vi "Operator Actions Log.vi"() -> (3 "?":string)   [LabVIEW 2017]
uses:
  <vilib>/OPCUA/NI OPC UA Client.lvlib
panel:
  in  "Stop Log":bool
  out "Operator Actions Recording":bool
  out "Log Loop":i32
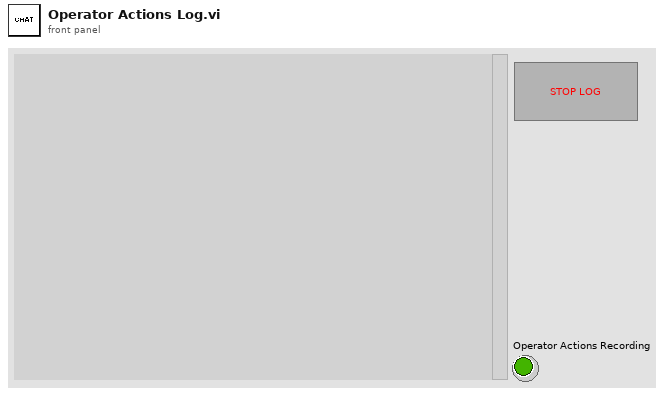
[diagram p1: front panel]
types:
  T1 = enum16{"open", "replace", "create", "open or create", "replace or create", "replace or create with confirmation"}
  T2 = typedef "OPC UA Client Refnum.ctl" = refnum<k21>
  T3 = typedef "Subscription ID.ctl" = u32
  T4 = typedef "Subscription Data Change.ctl" = cluster{"node ID":T5, " value":variant, "timestamp":timestamp, "data type":T6, "status code":T7}
  T5 = typedef "NodeId.ctl" = string
  T6 = typedef "Data Type.ctl" = u16
  T7 = typedef "OPC UA StatusCode.ctl" = u32
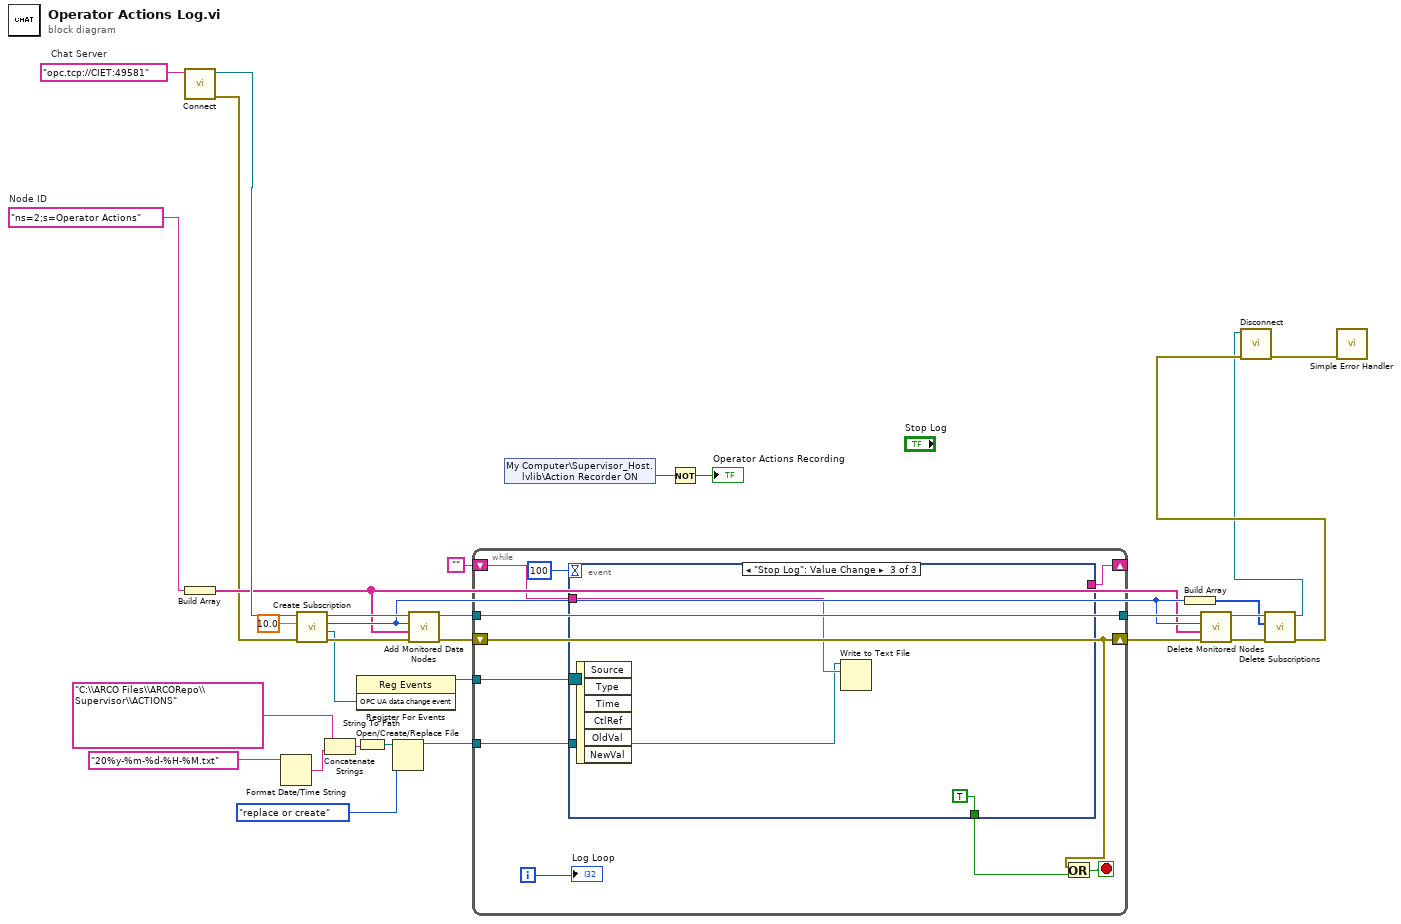
[diagram p0: block diagram]
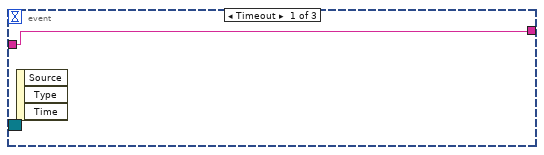
[diagram p2: hidden frame]
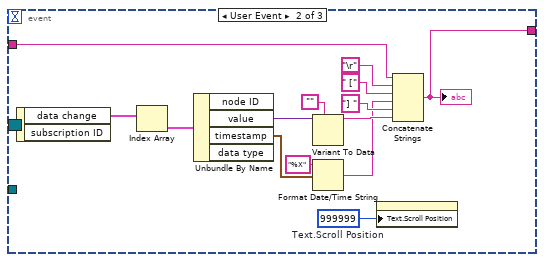
[diagram p3: hidden frame]
diagram:
  w15 = "ns=2;s=Operator Actions"  # Node ID
  w30 = "opc.tcp://CIET:49581"  # Chat Server
  n1 = call <vilib>:"Connect.vi"("server endpoint URL"=w30) -> ("error out"=w6:errorcluster, "OPC UA client refnum out"=w29:T2)  [unwired: 8 in, 1 out]
  n2 = Build Array(w15) -> (w14:string[])
  n3 = Format Date/Time String(time format string (%c)="20%y-%m-%d-%H-%M.txt") -> (date/time string=w10:string)  [unwired: 2 in]
  n4 = call <vilib>:"Create Subscription.vi"("error in (no error)"=w6, "publishing interval (1000 ms)"=10.0, "OPC UA client refnum in"=w29) -> ("error out"=w27:errorcluster, "OPC UA data change event"=w26:refnum<user-event>, "subscription ID out"=w18:T3, "OPC UA client refnum out"=w28:T2)  [unwired: 4 in, 1 out]
  n5 = Concatenate Strings("C:\\ARCO Files\\ARCORepo\\Supervisor\\ACTIONS", w10) -> (w8:string)
  n6 = register-events(w26) -> (reference out=w25:refnum<event-registration>)  [unwired: 2 in, 1 out]
  n7 = String To Path(string=w8) -> (path=w7:path)
  n8 = Open/Create/Replace File(file path (use dialog)=w7, operation (0:open)=T1."replace or create") -> (refnum out=w16:refnum<file>)  [unwired: 4 in, 2 out]
  n9 = call <vilib>:"Add Monitored Data Nodes.vi"("error in (no error)"=w27, "node IDs"=w14, "subscription ID in"=w18, "OPC UA client refnum in"=w28) -> ("error out"=w21:errorcluster, "OPC UA client refnum out"=w23:T2)  [unwired: 4 in, 2 out]
  n10 = while {
    tunnel: w25 -> [w41]
    shift-right: [w39] -> _
    shift-left: "" -> [w40]
    tunnel: w23 -> [w38]
    tunnel: [w38] -> w22
    tunnel: w16 -> [w37]
    shift-right: [w33] -> w5
    shift-left: w21 -> [w33]
    i -> [w36]
    stop <- w34 stop-if-true
    n11 = event shown="[2] \"Stop Log\": Value Change" {
      selector: w41 -> [_ _ _]
      dyn-events: _ -> [_ _ _]
      timeout: 100 -> [_ _ _]
      tunnel: w40 -> [w42 w45 w59]
      tunnel: [w42 w44 _] -> w39
      tunnel: w37 -> [_ _ w58]
      tunnel: [_ _ TRUE] -> w32
      event Timeout {
        n12 = event-data() -> ()  [unwired: 1 in, 3 out]
      }
      event User Event {
        w43 = u32 999999  # Text.Scroll Position
        n13 = event-data() -> ("data change"=w56:T4[])  [unwired: 1 in, 1 out]
        n14 = Index Array(array=w56) -> (element=w55:T4)  [unwired: 1 in]
        n15 = Unbundle By Name(w55) -> ("value"=w54:variant, "timestamp"=w52:timestamp)  [unwired: 2 out]
        n16 = Variant To Data(type="", Variant=w54) -> (data=w50:string)  [unwired: 1 in, 1 out]
        n17 = Format Date/Time String(time format string (%c)="%X", seconds (now)=w52) -> (date/time string=w48:string)  [unwired: 1 in]
        n18 = property class="Str"("Text.Scroll Position"=w43) -> ()  [unwired: 2 in, 2 out]
        n19 = Concatenate Strings(w45, "\r", " [", w48, "] ", w50) -> (w44:string)
        "?" <- w44
      }
      event "Stop Log": Value Change {
        n20 = event-data() -> ()  [unwired: 1 in, 6 out]
        n21 = Write to Text File(file (use dialog)=w58, text=w59) -> ()  [unwired: 2 in, 3 out]
      }
    }
    n22 = Or(x=w33, y=w32) -> (x .or. y?=w34:bool)
    "Log Loop" <- w36
  }
  n23 = shared-variable "My Computer\\Supervisor_Host.lvlib\\Action Recorder ON"() -> (w2:bool)  [unwired: 1 in, 1 out]
  n24 = Not(x=w2) -> (.not. x?=→"Operator Actions Recording":bool)
  n25 = Build Array(w18) -> (w17:T3[])
  n26 = call <vilib>:"Delete Monitored Nodes.vi"("error in (no error)"=w5, "node IDs"=w14, "subscription ID in"=w18, "OPC UA client refnum in"=w22) -> ("error out"=w19:errorcluster, "OPC UA client refnum out"=w20:T2)  [unwired: 3 in, 3 out]
  n27 = call <vilib>:"Delete Subscriptions.vi"("error in (no error)"=w19, "subscription IDs"=w17, "OPC UA client refnum in"=w20) -> ("error out"=w4:errorcluster, "OPC UA client refnum out"=w1:T2)  [unwired: 6 in, 1 out]
  n28 = call <vilib>:"Disconnect.vi"("error in (no error)"=w4, "OPC UA client refnum in"=w1) -> ("error out"=w31:errorcluster)  [unwired: 9 in]
  n29 = call <vilib>:"Simple Error Handler.vi"("error in (no error)"=w31) -> ()  [unwired: 4 in, 5 out]
